vi "prb2_sol.vi"() -> ()   [LabVIEW 2017]
panel:
  out "String":string
  in  "stop":bool
  in  "Path":path
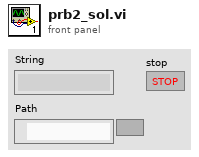
[diagram p1: front panel]
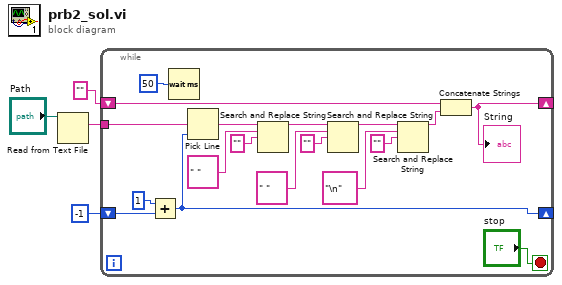
[diagram p0: block diagram]
diagram:
  n1 = Read from Text File(file (use dialog)="Path") -> (text=w2:string)  [unwired: 3 in, 3 out]
  n2 = while {
    shift-right: [w18] -> _
    shift-left: -1 -> [w19]
    tunnel: w2 -> [w17]
    shift-right: [w12] -> _
    shift-left: "" -> [w16]
    stop <- "stop" stop-if-true
    n3 = Add(x=1, y=w19) -> (x+y=w18:i32)
    n4 = Wait (ms)(milliseconds to wait=u32 50) -> ()  [unwired: 1 out]
    n5 = Pick Line(multi-line string=w17, line index=w18) -> (output string=w13:string)  [unwired: 1 in]
    n6 = Search and Replace String(input string=w13, search string=" ", replace string="") -> (result string=w6:string)  [unwired: 5 in, 3 out]
    n7 = Search and Replace String(input string=w6, search string=" ", replace string="") -> (result string=w5:string)  [unwired: 5 in, 3 out]
    n8 = Search and Replace String(input string=w5, search string="\n", replace string="") -> (result string=w9:string)  [unwired: 5 in, 3 out]
    n9 = Concatenate Strings(w16, w9) -> (w12:string)
    "String" <- w12
  }
